vi "CC Observation File Header.vi"(8 "error in (no error)":errorcluster) -> (0 "error out":errorcluster, 3 "Header":string[](array[string]))   [LabVIEW 2024]
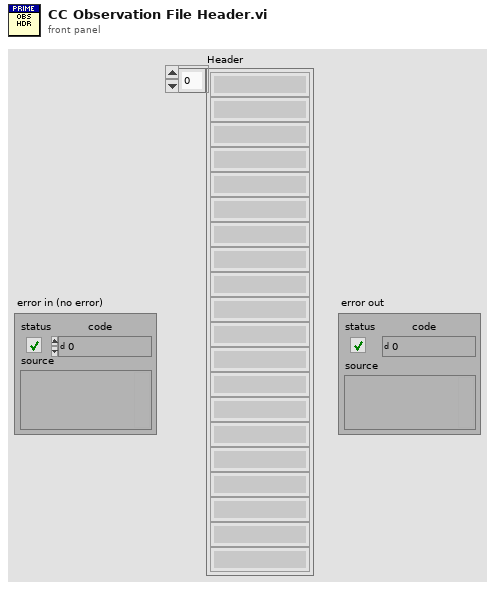
[diagram p1: front panel]
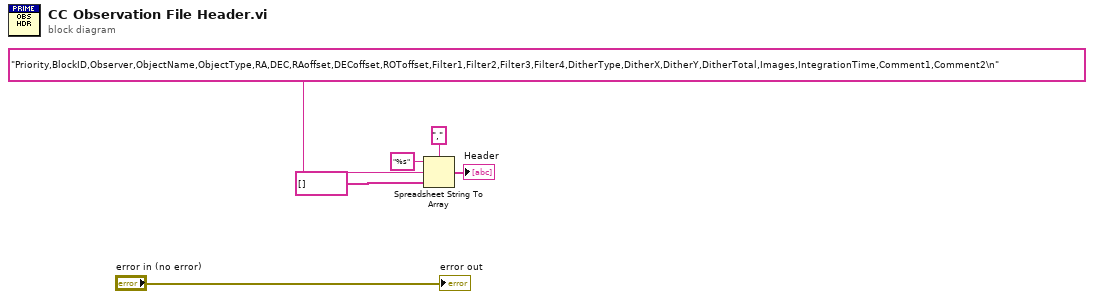
[diagram p0: block diagram]
diagram:
  n1 = Spreadsheet String To Array(delimiter (Tab)=",", format string="%s", spreadsheet string="Priority,BlockID,Observer,ObjectName,ObjectType,RA,DEC,RAoffset,DECoffset,ROToffset,Filter1,Filter2,Filter3,Filter4,DitherType,DitherX,DitherY,DitherTotal,Images,IntegrationTime,Comment1,Comment2\n", array type (2D Dbl)=string[] []) -> (array=→"Header":string[])
  "error out" <- "error in (no error)"
